vi "SubVI_Grab_Optimal_Model_params.vi"(11 "Optimal Model Parameters":T2) -> (2 "Window Size":i32, 3 "Zeros Array with window size":dbl[][](array[numeric]), 4 "Covariance Matrix":dbl[][](array[numeric]), 5 "Time Window":dbl[](array[numeric]), 6 "GO Epoch Means":dbl[](array[numeric]), 9 "Hyperparameters":T1)   [LabVIEW 2020]
uses:
  <vilib>/Analysis/Matrix/Numeric/Conversions/Matrix To Array - RM.vi
  <vilib>/gmath/NI_Gmath.lvlib
  <vilib>/Analysis/Matrix/NI_Matrix.lvlib
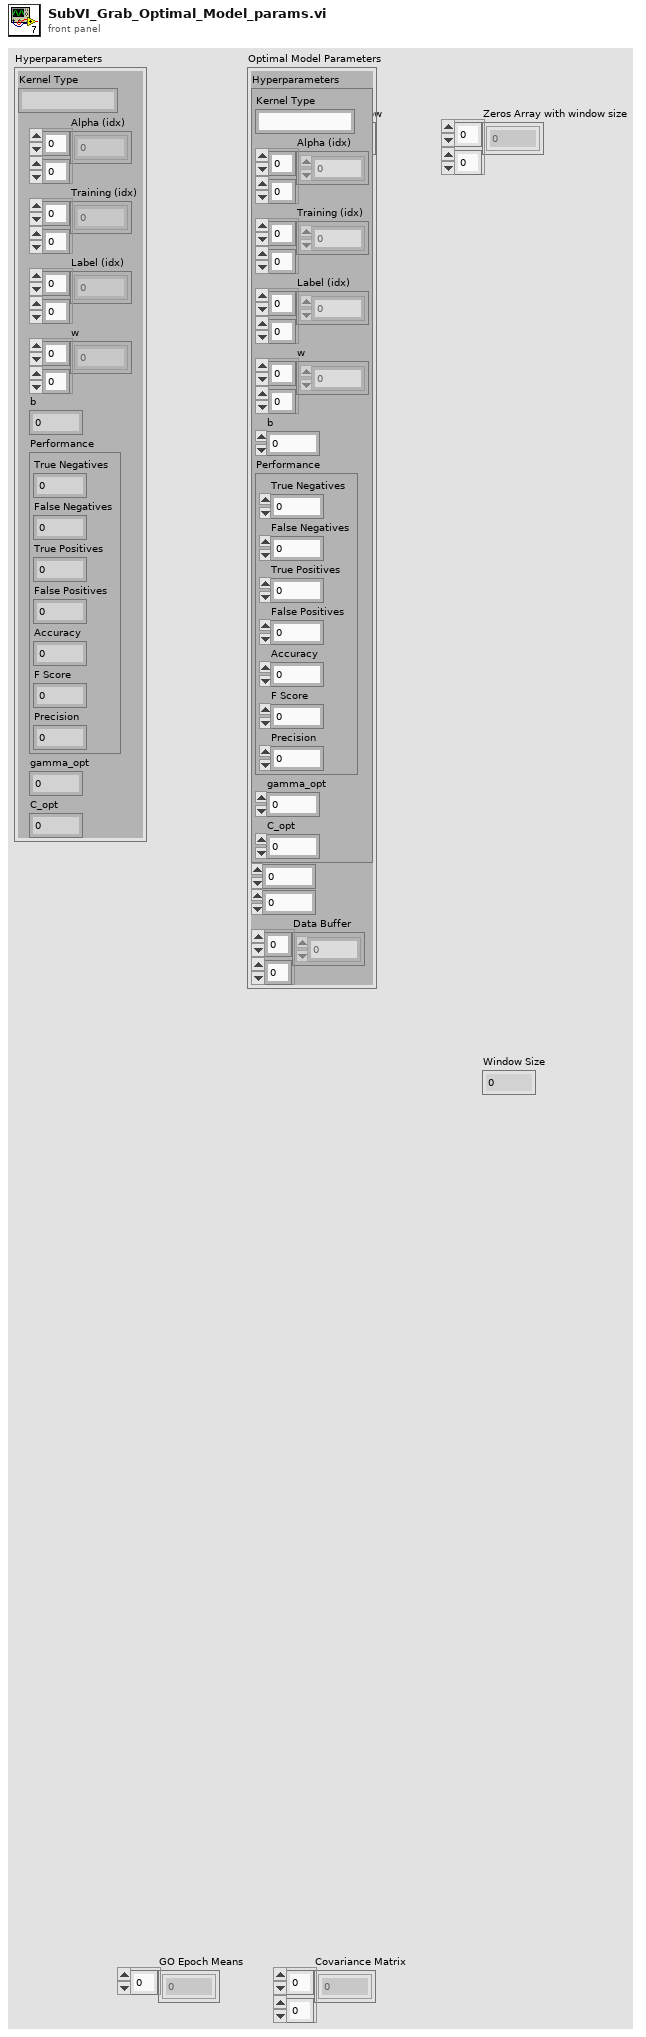
[diagram p1: front panel]
types:
  T1 = cluster{"Kernel Type":string, "Alpha (idx)":dbl[][], "Training (idx)":dbl[][], "Label (idx)":dbl[][], "w":dbl[][], "b":dbl, "Performance":cluster{"True Negatives":i32, "False Negatives":i32, "True Positives":i32, "False Positives":i32, "Accuracy":dbl, "F Score":dbl, "Precision":dbl}, "gamma_opt":dbl, "C_opt":dbl}
  T2 = cluster{"Hyperparameters":cluster{"Kernel Type":string, "Alpha (idx)":dbl[][], "Training (idx)":dbl[][], "Label (idx)":dbl[][], "w":dbl[][], "b":dbl, "Performance":cluster{"True Negatives":i32, "False Negatives":i32, "True Positives":i32, "False Positives":i32, "Accuracy":dbl, "F Score":dbl, "Precision":dbl}, "gamma_opt":dbl, "C_opt":dbl}, i32, dbl, "Data Buffer":dbl[][]}
  T3 = typedef "NI_Matrix.lvlib/RealMatrix.ctl" = dbl[][]
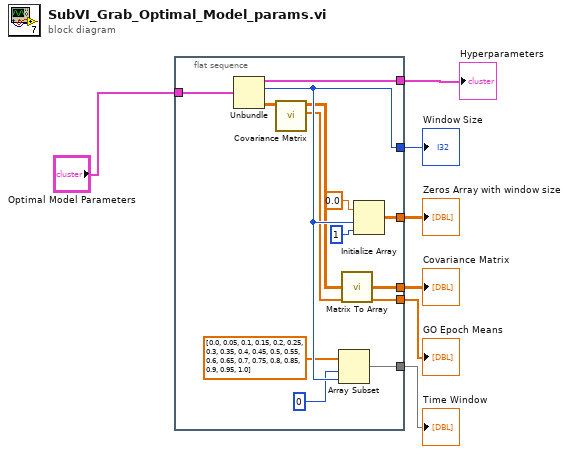
[diagram p0: block diagram]
diagram:
  n1 = flat-sequence {
    tunnel: [w20] -> w3
    tunnel: [w19] -> w4
    tunnel: [w18] -> w5
    tunnel: [w17] -> w6
    tunnel: [w14] -> w1
    tunnel: [w13] -> w7
    tunnel: "Optimal Model Parameters" -> [w12]
    frame #0 {
      n2 = Unbundle(w12) -> ("Hyperparameters"=w14:T1, w19:i32, "Data Buffer"=w16:dbl[][])  [unwired: 1 out]
      n3 = call <vilib>:"Covariance Matrix.vi"("X"=w16) -> ("mean vector"=w17:dbl[], "covariance matrix V"=w15:T3)  [unwired: 9 in]
      n4 = Array Subset(array=dbl[] [0.0, 0.05, 0.1, 0.15, 0.2, 0.25, 0.3, 0.35, 0.4, 0.45, 0.5, 0.55, 0.6, 0.65, 0.7, 0.75, 0.8, 0.85, 0.9, 0.95, 1.0] ("Sliding_window"), index=0, length=w19) -> (w20:dbl[])
      n5 = call-poly <vilib>:"Matrix To Array.vi"("Real Matrix"=w15) -> ("Real 2D Array"=w18:dbl[][])
      n6 = Initialize Array(0.0 ("element"), w19, 1 ("dimension size")) -> (w13:dbl[][])
    }
  }
  "Zeros Array with window size" <- w7
  "GO Epoch Means" <- w6
  "Covariance Matrix" <- w5
  "Window Size" <- w4
  "Time Window" <- w3
  "Hyperparameters" <- w1
